vi "Collect Signals.vi"() -> ()   [LabVIEW 2011]
doc: "This example shows how to use the Collector Express VI. The Collector Express VI collects and returns input signals. You can specify the maximum number of samples the Collector can hold. When you call this Express VI repeatedly, as the While Loop in this example does, and the Express VI reaches the maximum number of samples per channel, the Express VI discards the oldest data and adds the newest data to the collected samples. This example shows the differences in collected data when you change the maximum number of samples.\n\n1. Run the VI. The Collector is configured to hold a maximum of 450 samples. Since the input signal transmits 100 samples to the Collector each time the While Loop executes, it takes five loop iterations for the Collector to receive the maximum number of samples. In the fifth iteration, the Collector starts discarding old data as new data arrives. However, because the maximum number of samples the Collector can hold is greater than the samples received in each loop iteration, the output graph for the Collector VI still contains data from previous loop iterations.\n\n2. Stop the VI. On the block diagram, double-click the Collector Express VI to open the <B>Configure Collector</B> dialog box and change the <B>Maximum number of samples</B> from 450 to 50. Close the dialog box and run the VI again. The input signal still transmits 100 samples to the Collector in each loop iteration, but the Collector now holds a maximum of only 50 samples. Thus, each time the loop iterates, the Collector holds only the 50 most recent samples and discards the 50 previous samples. In this case, the Collector does not hold data from previous loop iterations because it collects the maximum number of samples in each iteration."
uses:
  Instance           3 23Saved   Collect Signals .vi
  Instance           2 23Saved   Collect Signals .vi
  Instance           1 23Saved   Collect Signals .vi
panel:
  out "Input Signals":dynamicdata(graph) caption="Collected Signals"
  in  "stop":bool
  out "Collected Signals":dynamicdata(graph)
  # "Select Help»Show Context Help and move the cursor over the VI icon to display help for this VI."
  # "Instructions:\n\n1. Run the VI. The Collector is configured to hold a maximum of 450 samples. Since the input signal transmits 100 samples each time the While Loop executes, it takes five loop iterations for the Collector to receive the maximum number of samples. In the fifth iteration, the Collector starts discarding old data as new data arrives. However, because the maximum number of samples is greater than the samples received in each loop iteration, the output graph for the Collector VI still contains data from previous loop iterations.\n\n\n2. Stop the VI. On the block diagram, double-click the Collector Express VI to open the Configure Collector dialog box and change the Maximum number of samples from 450 to 50. Close the dialog box and run the VI again. The input signal still transmits 100 samples to the Collector in each loop iteration, but the Collector now holds a maximum of only 50 samples. Thus, each time the loop iterates, the Collector holds only the 50 most recent samples and discards the 50 previous samples. In this case, the Collector does not hold data from previous loop iterations because it collects the maximum number of samples in each iteration."
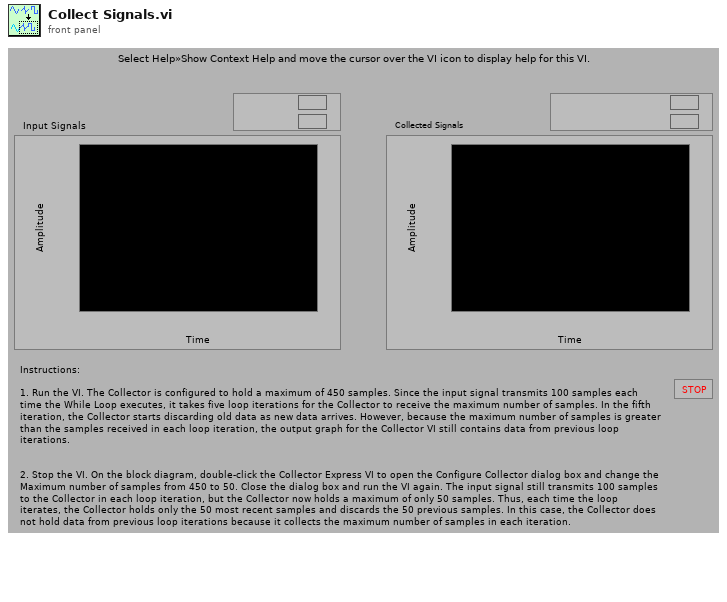
[diagram p1: front panel]
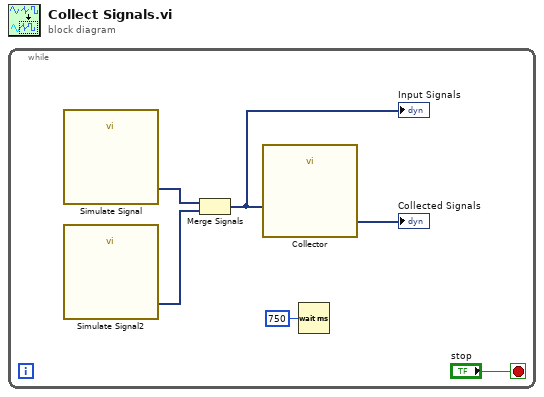
[diagram p0: block diagram]
diagram:
  n1 = while {
    stop <- "stop" stop-if-true
    n2 = call "Simulate Signal"() -> ("Sine"=w3:dynamicdata)  [unwired: 14 in, 1 out]
    n3 = call "Simulate Signal2"() -> ("Triangle"=w1:dynamicdata)  [unwired: 14 in, 1 out]
    n4 = Merge Signals(w3, w1) -> (w2:dynamicdata)
    "Input Signals" <- w2
    n5 = call "Collector"("Signals"=w2) -> ("Collected Signals"=→"Collected Signals":dynamicdata)  [unwired: 9 in, 1 out]
    n6 = Wait (ms)(milliseconds to wait=u32 750 ("millisecond multiple")) -> ()  [unwired: 1 out]
  }
